vi "TSCAN_SetData.vi"(8 "错误输入（无错误）":errorcluster, 9 "CAN配置":T1={"硬件类型"=8, "硬件子类型"=0, "ABaudrateKbps"=250.0, "AListenOnly"=enum."Normal", "Int120Ohm"=enum."Enable", "EnableChannel"=enum."Enable", "AHwChannel"=0, "AAppChannel"=0} {"AAppChannel" items=["CHN1", "CHN2", "CHN3", "CHN4", "CHN5", "CHN6", "CHN7", "CHN8", "CHN9", "CHN10", "CHN11", "CHN12", "CHN13", "CHN14", "CHN15", "CHN16", "CHN17", "CHN18", "CHN19", "CHN20", "CHN21", "CHN22", "CHN23", "CHN24", "CHN25", "CHN26", "CHN27", "CHN28", "CHN29", "CHN30", "CHN31", "CHN32"]; "AHwChannel" items=["CHN1", "CHN2", "CHN3", "CHN4", "CHN5", "CHN6", "CHN7", "CHN8", "CHN9", "CHN10", "CHN11", "CHN12", "CHN13", "CHN14", "CHN15", "CHN16", "CHN17", "CHN18", "CHN19", "CHN20", "CHN21", "CHN22", "CHN23", "CHN24", "CHN25", "CHN26", "CHN27", "CHN28", "CHN29", "CHN30", "CHN31", "CHN32"]; "硬件子类型" items=["BUS_UNKNOWN_TYPE", "TSCAN_PRO_4", "TSCAN_LITE_2", "TSCANMini", "TSLinMini", "TSCANFDmini", "TSCAN_LIN_IO_2", "TSCAN_LITE_2", "TSCANLIN", "TSCAN_FD_Mini_1"]; "硬件类型" items=["BUS_UNKNOWN_TYPE", "TS_TCP_DEVICE", "XL_USB_DEVICE", "TS_USB_DEVICE", "PEAK_USB_DEVICE", "KVASER_USB_DEVICE", "ZLG_USB_DEVICE", "ICS_USB_DEVICE", "TS_TC1005_DEVICE"]}, 11 "路径输入":path) -> (0 "错误输出":errorcluster, 2 "AAPPChannel":i32, 3 "路径输出":path, 4 "Set_Baudrated_Successfully":bool, 6 "Mapping_Successfully":bool)   [LabVIEW 2019]
panel:
  # "用N路can通道，设置N路CAN通道"
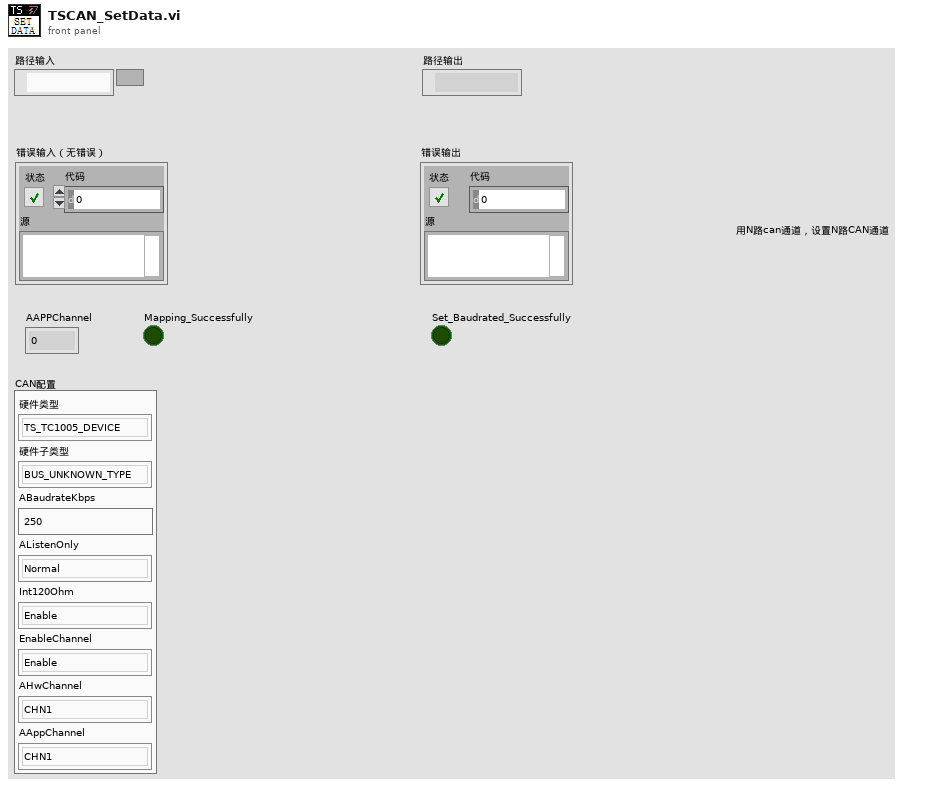
[diagram p1: front panel]
types:
  T1 = cluster{"硬件类型":i32, "硬件子类型":i32, "ABaudrateKbps":sgl, "AListenOnly":enum16{"Normal", "ListenOnly"}, "Int120Ohm":enum16{"Disable", "Enable"}, "EnableChannel":enum16{"Disable", "Enable"}, "AHwChannel":i32, "AAppChannel":i32}
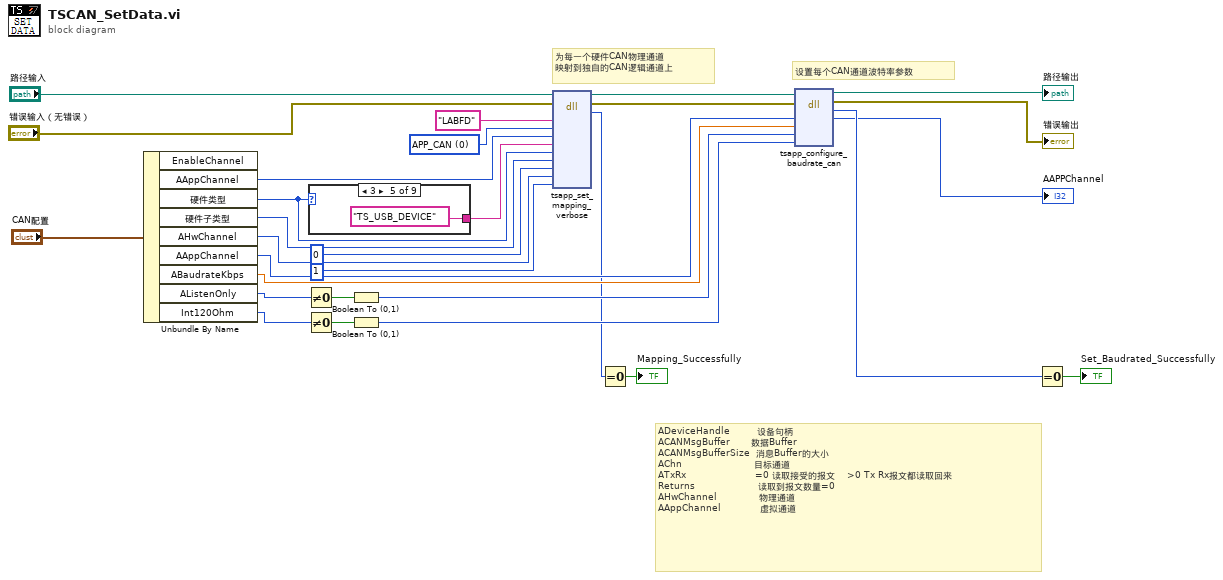
[diagram p0: block diagram]
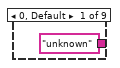
[diagram p2: hidden frame]
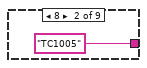
[diagram p3: hidden frame]
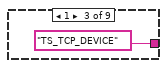
[diagram p4: hidden frame]
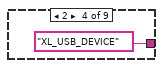
[diagram p5: hidden frame]
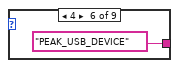
[diagram p6: hidden frame]
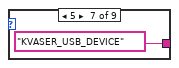
[diagram p7: hidden frame]
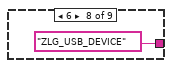
[diagram p8: hidden frame]
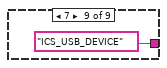
[diagram p9: hidden frame]
diagram:
  w27 = 0 items=["APP_CAN", "APP_LIN"] ("AAppChannelType")
  # "ADeviceHandle         设备句柄\nACANMsgBuffer       数据Buffer\nACANMsgBufferSize  消息Buffer的大小\nAChn                        目标通道\nATxRx                       =0 读取接受的报文    >0 Tx Rx报文都读取回来\nReturns                     读取到报文数量=0\nAHwChannel              物理通道\nAAppChannel             虚拟通道"
  # "设置每个CAN通道波特率参数"
  # "为每一个硬件CAN物理通道\n映射到独自的CAN逻辑通道上"
  n1 = Unbundle By Name("CAN配置") -> ("AAppChannel"=w26:i32, "硬件类型"=w24:i32, "硬件子类型"=w23:i32, "AHwChannel"=w21:i32, "AAppChannel"=w19:i32, "ABaudrateKbps"=w18:sgl, "AListenOnly"=w15:enum16{"Normal", "ListenOnly"}, "Int120Ohm"=w13:enum16{"Disable", "Enable"})  [unwired: 1 out]
  n2 = Not Equal To 0?(x=w15) -> (x != 0?=w17:bool)
  n3 = Not Equal To 0?(x=w13) -> (x != 0?=w16:bool)
  n4 = case shown="3" w24 {
    tunnel: ["unknown" ("AHardwareName") "TC1005" ("AHardwareName") "TS_TCP_DEVICE" ("AHardwareName") "XL_USB_DEVICE" ("AHardwareName") "TS_USB_DEVICE" ("AHardwareName") "PEAK_USB_DEVICE" ("AHardwareName") "KVASER_USB_DEVICE" ("AHardwareName") "ZLG_USB_DEVICE" ("AHardwareName") "ICS_USB_DEVICE" ("AHardwareName")] -> w25
    frame 0, Default {
    }
    frame 8 {
    }
    frame 1 {
    }
    frame 2 {
    }
    frame 3 {
    }
    frame 4 {
    }
    frame 5 {
    }
    frame 6 {
    }
    frame 7 {
    }
  }
  n5 = Boolean To (0,1)(Boolean=w17) -> (0, 1=w14:i16)
  n6 = Boolean To (0,1)(Boolean=w16) -> (0, 1=w12:i16)
  n7 = dll-call lib="PTH2Habs CUsers\nAdministratorDesktopTS_Can通讯PathTSMaster.dll" fn="tsapp_set_mapping_verbose"(path in="路径输入", error in="错误输入（无错误）", "FAPppName"="LABFD" ("AppName"), "AChnType"=w27, "FAppChannelIndex"=w26, "AHWDeviceName"=w25, "AHWDeviceType"=w24, "AHWDeviceSubType"=w23, "AldHW"=0, "AldHWChn"=w21, "FMappingDisabled"=u32 1) -> (path out=w29:path, error out=w6:errorcluster, "tsapp_set_mapping_verbose"=w8:i32)  [unwired: 10 in]
  n8 = Equal To 0?(x=w8) -> (x = 0?=→"Mapping_Successfully":bool)
  n9 = dll-call lib="PTH2Habs CUsers\nAdministratorDesktopTS_Can通讯PathTSMaster.dll" fn="tsapp_configure_baudrate_can"(path in=w29, error in=w6, "ALdxChn"=w19, "ABaudrateKbps"=w18, "AlistenOnly"=w14, "AlnstallTermResistor120Ohm"=w12) -> (path out=→"路径输出":path, error out=→"错误输出":errorcluster, "tsapp_configure_baudrate_can"=w9:i32, "ALdxChn"=→"AAPPChannel":i32)  [unwired: 4 in]
  n10 = Equal To 0?(x=w9) -> (x = 0?=→"Set_Baudrated_Successfully":bool)
